vi "tio32_Open.vi"(5 "error in (no error)":errorcluster, 8 "VISA resource name":refnum<visa-resource-name>) -> (0 "error out":errorcluster, 2 "return":i32=666, 3 "VISA resource name out":refnum<visa-resource-name>)   [LabVIEW 2011]
doc: "DLL tio32.dll\nFunction INT16TYPE WINAPI tio32_Open(void);\n\nInitialize the DLL."
uses:
  l_pse_dll/Tio32.dll
panel:
  # "tio32_Open"
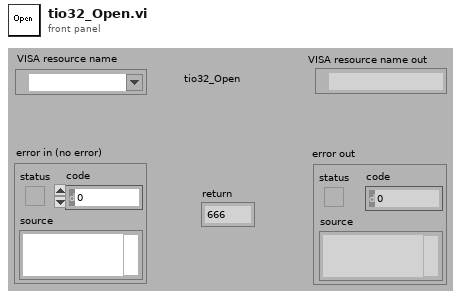
[diagram p1: front panel]
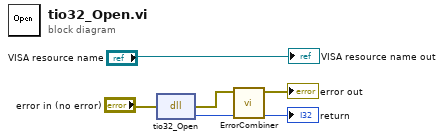
[diagram p0: block diagram]
diagram:
  n1 = dll-call lib="C:/Users/Ikaika's/Documents/DCC/Apps/INA231/INA231-SFT-rev1/INA231-Sourcecode-rev1/INA231/Shell Resources/l_pse_dll/Tio32.dll" fn="tio32_Open"(error in="error in (no error)") -> (error out=w1:errorcluster, "Rückgabetyp"=w3:i32)  [unwired: 2 in, 1 out]
  n2 = call "ErrorCombiner.vi"("Return In"=w3, "error in (no error)"=w1) -> ("Return Out"=→"return":i32, "error out"=→"error out":errorcluster)  [unwired: 8 in]
  "VISA resource name out" <- "VISA resource name"
